vi "Go to Move.vi"(8 "Error In":errorcluster, 9 "Absolute Y":dbl, 10 "Absolute X":dbl, 11 "Address/Port in":i16) -> (0 "Error Out":errorcluster, 3 "Address/Port out":i16)   [LabVIEW 2014]
doc: "Move the motors \"X\" and \"Y\" to the absolute positions Absolute X and Absolute Y. Final positions depends on the Origin set on the motors"
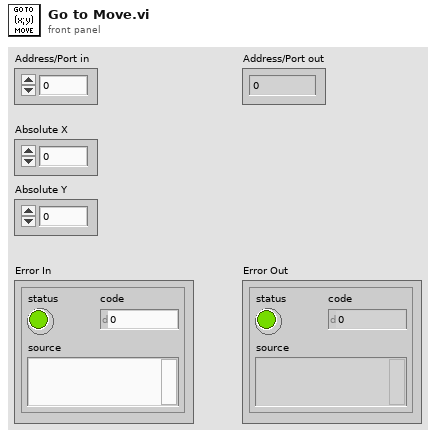
[diagram p1: front panel]
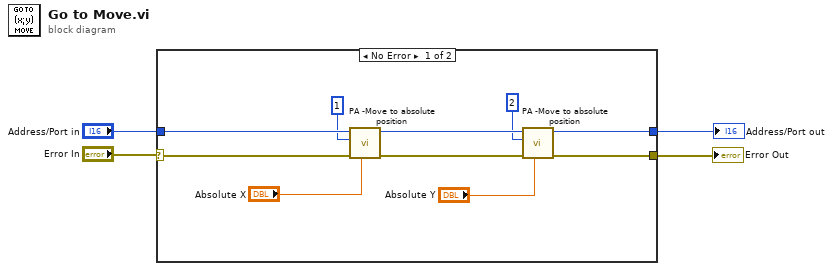
[diagram p0: block diagram]
diagram:
  n1 = case shown="No Error" "Error In" {
    selector: "Error In" -> [w13 w16]
    tunnel: [w8 w16] -> w3
    tunnel: "Address/Port in" -> [w14 w15]
    tunnel: [w7 w15] -> w1
    frame No Error {
      n2 = call "PA -Move to absolute position.vi"("Move to absolute\nposition - set"="Absolute X", "error in"=w13, "Axis #"=i8 1 ("Axis  #"), "Address / Port"=w14) -> ("error out"=w11:errorcluster, "Address / Port dup"=w10:i16)  [unwired: 2 in, 2 out]
      n3 = call "PA -Move to absolute position.vi"("Move to absolute\nposition - set"="Absolute Y", "error in"=w11, "Axis #"=i8 2 ("Axis  #"), "Address / Port"=w10) -> ("error out"=w8:errorcluster, "Address / Port dup"=w7:i16)  [unwired: 2 in, 2 out]
    }
    frame Error {
    }
  }
  "Error Out" <- w3
  "Address/Port out" <- w1
